vi "transfer char run_subvi_05_11a_JW.vi"(0 "VISA session":refnum<visa-resource-name>="GPIB0::17::INSTR", 5 "Var1 sweep settings":T4={"start"=40.0, "stop"=-40.0, "step (linear only)"=-1.0, "sweep spacing (linear: 0)"=0, "sweep mode"=FALSE, "compliance (V)"=100.0, "compliance (A)"=0.001} {"compliance (A)" format="%^.2e"; "compliance (V)" format="%.2f"; "sweep spacing (linear: 0)" items=["linear", "log 10", "log 25", "log 50"]; "step (linear only)" format="%.2f"; "stop" format="%.2f"; "start" format="%.2f"}, 7 "Var2 step settings":T3={"compliance (A)"=0.001, "compliance (V)"=100.0, "start"=-2.0, "total points"=2, "step"=-38.0} {"step" format="%.2f"; "start" format="%.2f"; "compliance (V)" format="%.2f"; "compliance (A)" format="%^.2e"}, 9 "integration time":u32(slide) scale=0.0..2.0, 11 "Input Path":path, 13 "Sample Properties:":T1 {"Date Created" format="%<%x>T"}) -> (1 "Trap Density-STS":dbl, 3 "Trap Density-VT":dbl, 4 "Mobility":dbl, 6 "graphic display":cluster{"trace":dbl[], "trace":dbl[]}(graph), 8 "On/Off Current":dbl, 10 "XY Graph":cluster{dbl[], "trace":dbl[]}[](graph), 12 "Vt":dbl, 14 "STS":dbl, 15 "error?":errorcluster)   [LabVIEW 2011]
uses:
  <vilib>/Utility/file.llb/Write To Spreadsheet File (DBL).vi
  <vilib>/Utility/file.llb/Read From Spreadsheet File (string).vi
  <vilib>/Utility/file.llb/Write To Spreadsheet File (string).vi
  <vilib>/Analysis/NI_AALPro.lvlib
panel:
  out "Array":string[][](array[string])
  in  "Output Path":path
  in  "Temp (K)":dbl=0.001 format="%^.2e"
  in  "NumPts":dbl=5.0
  out "Numeric":dbl
  out "Max R":i32[](listbox)
  out "min r":dbl
  out "max r":dbl
  out "error? 2":errorcluster
  in  "MAXIMUM":ext format="%.2e"
  in  "MINIMUM":ext=-1e-05 format="%_2e"
  out "graphic display 2":cluster{"trace":dbl[], "trace":dbl[]}(graph)
  in  "Y1 axis":string="Id"
  in  "Y2 axis settings":T2 {"MAXIMUM" format="%.9f"; "MINIMUM" format="%.9f"}
  in  "wait time parameter":dbl=1.0
  in  "Value (Either V or A) 4":dbl
  in  "Value (Either V or A) 3":dbl
  in  "Value (Either V or A) 2":dbl
  in  "Value (V or A)":dbl
  in  "compliance (A)":dbl=0.001 format="%^.2e"
  in  "compliance (V)":dbl=100.0 format="%^.2e"
  in  "Iname":string="Is"
  in  "Vname":string="Vs"
  in  "Function":u16(ring)=4 items=["disabled", "Var1", "Var2", "Var1'", "Constant"]
  in  "Mode":u16(ring)=4 items=["V", "I", "VPulse", "IPulse", "Common"]
  in  "Iname 4":string="I4"
  in  "Vname 4":string="V4"
  in  "Function 4":u16(ring)=4 items=["disabled", "Var1", "Var2", "Var1'", "Constant"]
  in  "Mode 4":u16(ring) items=["V", "I", "VPulse", "IPulse", "Common"]
  in  "Iname 3":string="Ig"
  in  "Vname 3":string="Vg"
  in  "Function 3":u16(ring)=1 items=["disabled", "Var1", "Var2", "Var1'", "Constant"]
  in  "Mode 3":u16(ring) items=["V", "I", "VPulse", "IPulse", "Common"]
  in  "Iname 2":string="Id"
  in  "Vname 2":string="Vd"
  in  "Function 2":u16(ring)=2 items=["disabled", "Var1", "Var2", "Var1'", "Constant"]
  in  "Mode 2":u16(ring) items=["V", "I", "VPulse", "IPulse", "Common"]
  in  "reset":bool=TRUE
  # "SMU1"
  # "SMU2"
  # "SMU3"
  # "SMU4"
  # "Sample Properties:"
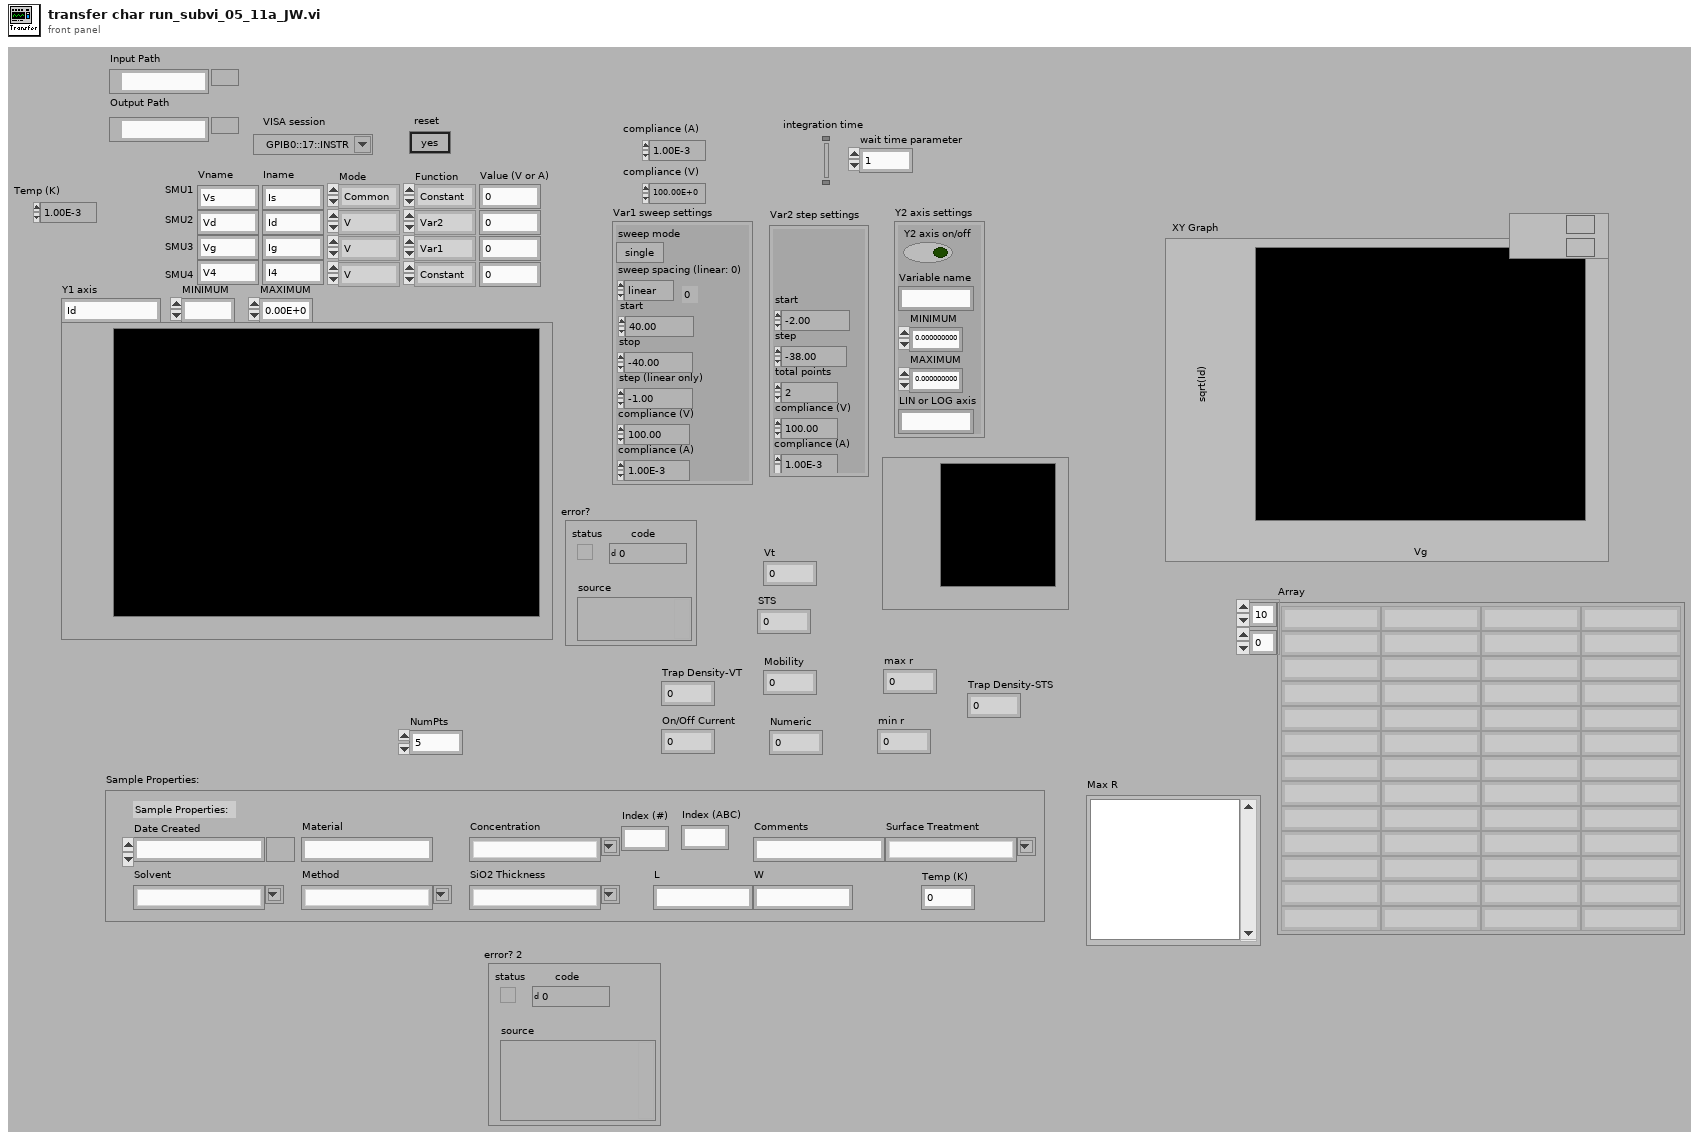
[diagram p1: front panel]
types:
  T1 = cluster{"Date Created":timestamp, "Material":string, "Solvent":string, "Concentration":string, "Method":string, "SiO2 Thickness":string, "Index (#)":string, "Index (ABC)":string, "L":string, "W":string, "Surface Treatment":string, "Comments":string, "Temp (K)":dbl}
  T2 = cluster{"Y2 axis on/off":bool, "MINIMUM":ext, "MAXIMUM":ext, "Variable name":string, "LIN or LOG axis":string}
  T3 = cluster{"compliance (A)":dbl, "compliance (V)":dbl, "start":dbl, "total points":u16, "step":dbl}
  T4 = cluster{"start":dbl, "stop":dbl, "step (linear only)":dbl, "sweep spacing (linear: 0)":u16, "sweep mode":bool, "compliance (V)":dbl, "compliance (A)":dbl}
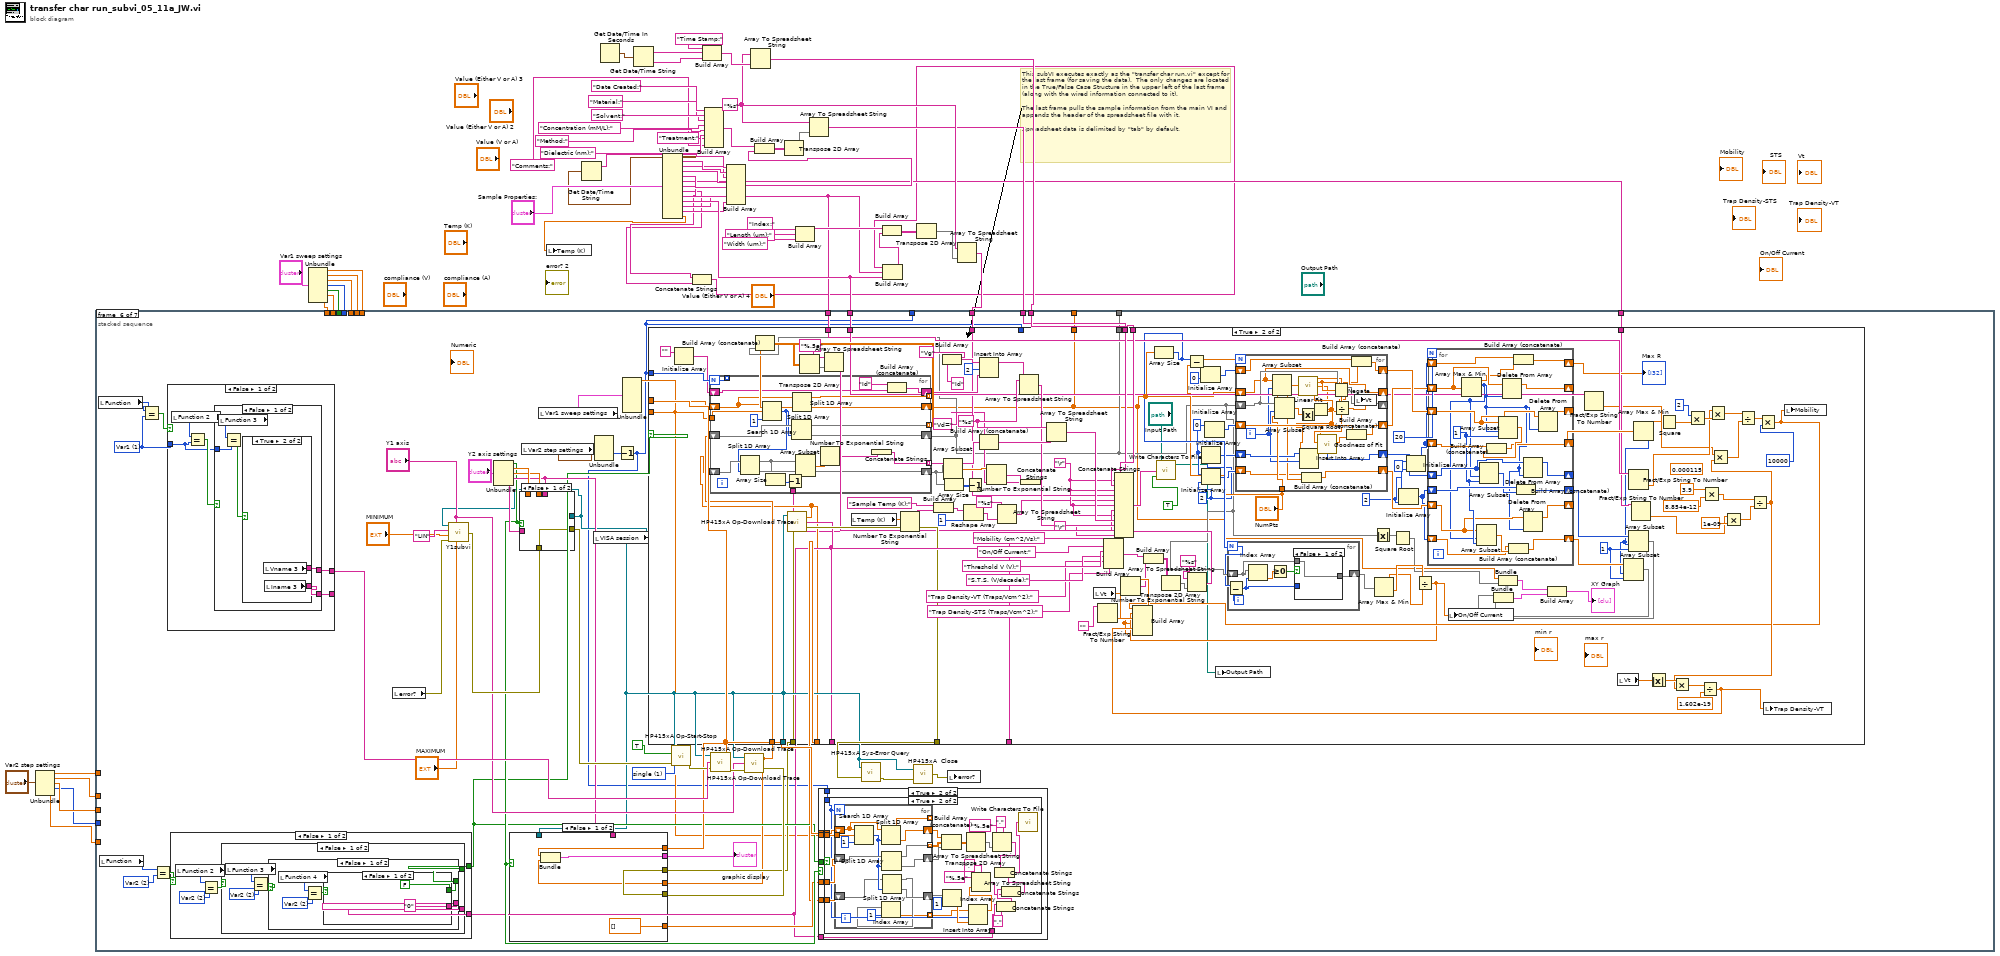
[diagram p0: block diagram]
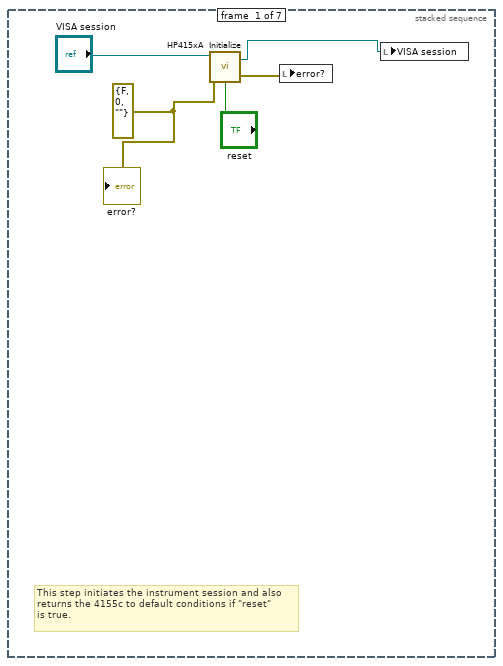
[diagram p2: hidden frame]
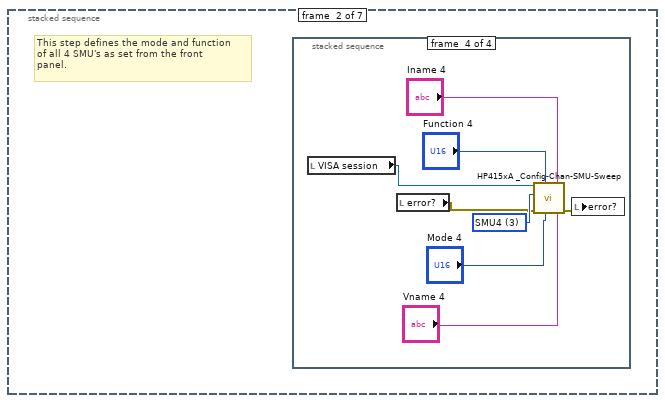
[diagram p3: hidden frame]
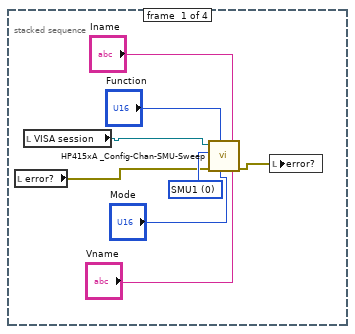
[diagram p4: hidden frame]
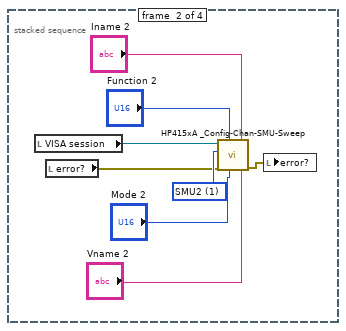
[diagram p5: hidden frame]
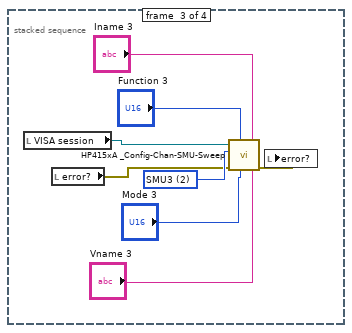
[diagram p6: hidden frame]
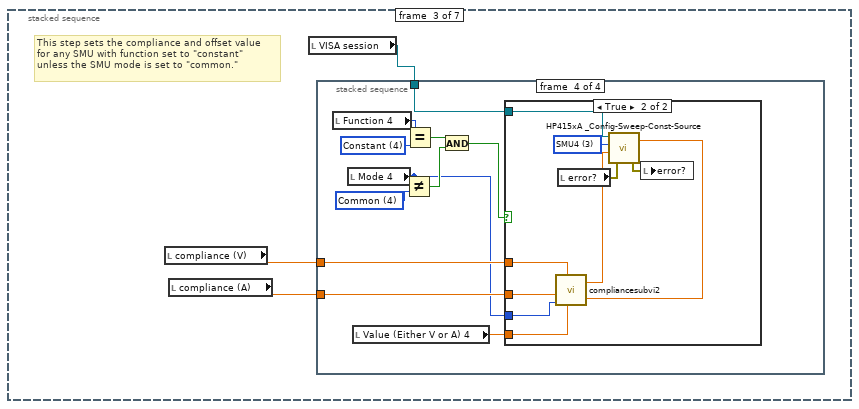
[diagram p7: hidden frame]
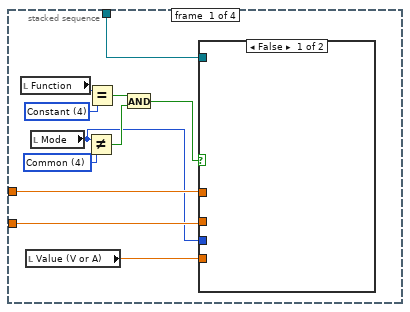
[diagram p8: hidden frame]
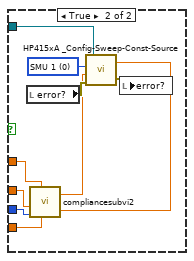
[diagram p9: hidden frame]
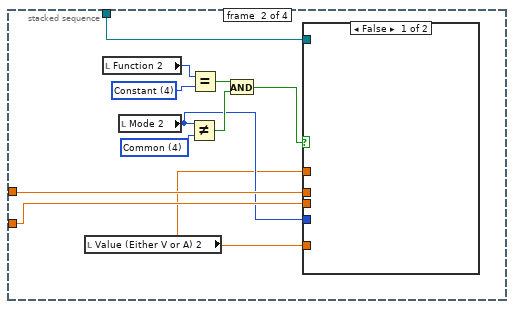
[diagram p10: hidden frame]
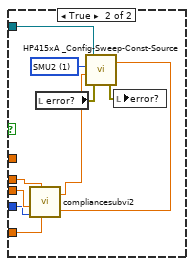
[diagram p11: hidden frame]
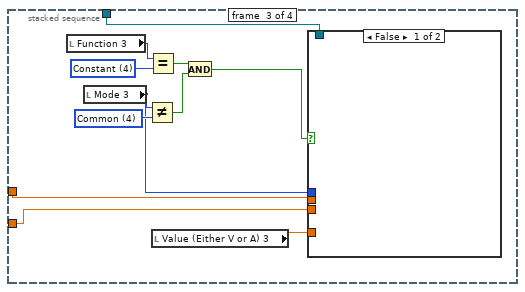
[diagram p12: hidden frame]
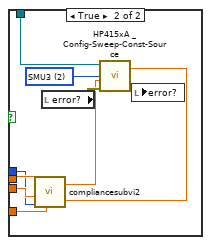
[diagram p13: hidden frame]
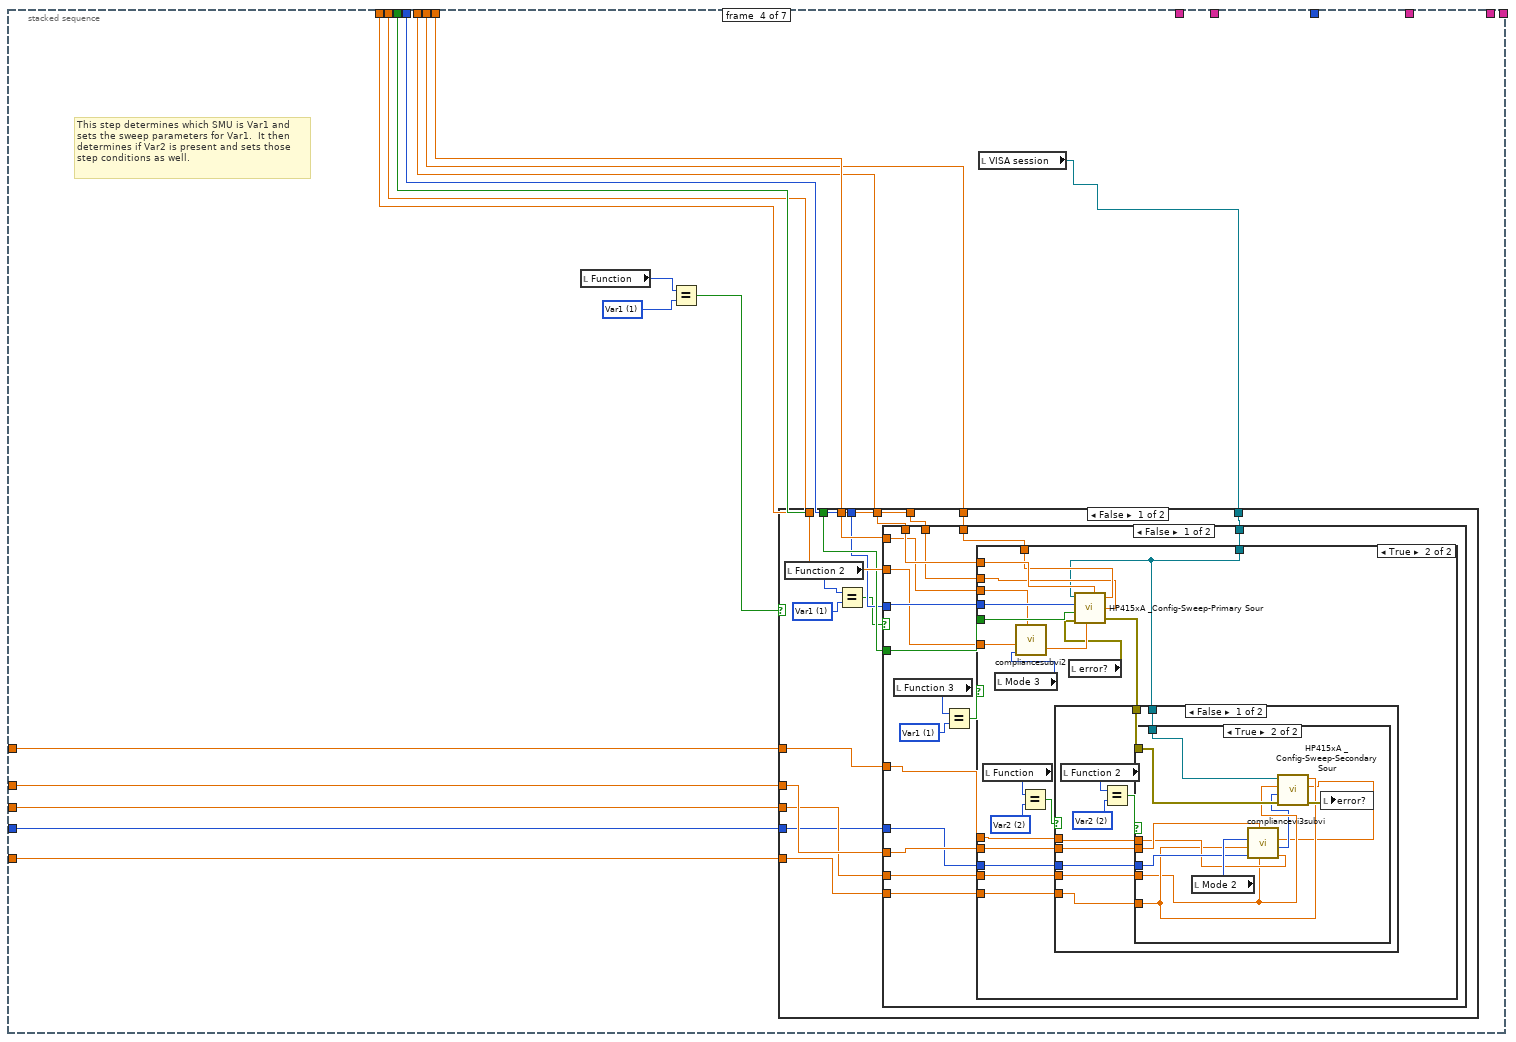
[diagram p15: hidden frame]
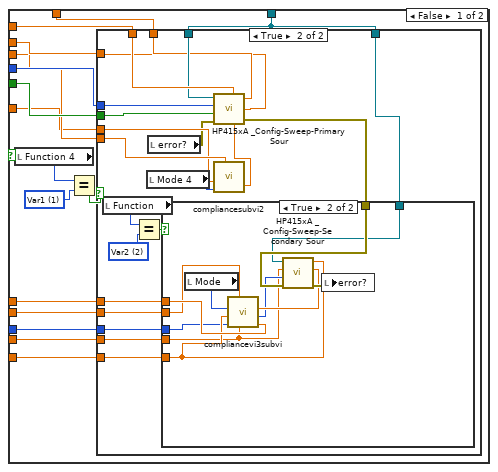
[diagram p16: hidden frame]
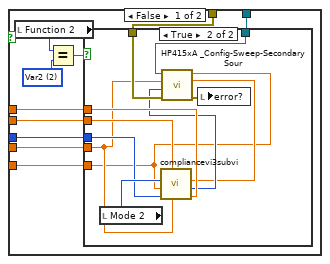
[diagram p18: hidden frame]
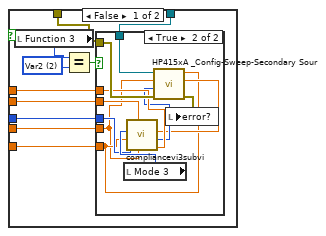
[diagram p19: hidden frame]
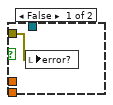
[diagram p20: hidden frame]
diagram:
  w31 = "%s"
  # "This subVI executes exactly as the \"transfer char run.vi\" except for the last frame (for saving the data).  The only changes are located in the True/False Case Structure in the upper left of the last frame (along with the wired information connected to it). \n\nThe last frame pulls the sample information from the main VI and appends the header of the spreadsheet file with it.\n\nSpreadsheet data is delimited by \"tab\" by default."
  n1 = Unbundle("Var2 step settings") -> ("compliance (A)"=w49:dbl, "compliance (V)"=w48:dbl, "start"=w47:dbl, "total points"=w46:u16, "step"=w45:dbl)
  n2 = Unbundle("Var1 sweep settings") -> ("start"=w57:dbl, "stop"=w56:dbl, "step (linear only)"=w55:dbl, "sweep spacing (linear: 0)"=w54:u16, "sweep mode"=w53:bool, "compliance (V)"=w52:dbl, "compliance (A)"=w51:dbl)
  n3 = Get Date/Time In Seconds() -> (seconds since 1Jan1904=w38:timestamp)
  n4 = Get Date/Time String(seconds (now)=w38) -> (date string=w37:string, time string=w36:string)  [unwired: 2 in]
  n5 = Unbundle("Sample Properties:") -> ("Date Created"=w16:timestamp, "Material"=w15:string, "Solvent"=w11:string, "Concentration"=w10:string, "Method"=w14:string, "SiO2 Thickness"=w9:string, "Index (#)"=w4:string, "Index (ABC)"=w3:string, "L"=w7:string, "W"=w8:string, "Surface Treatment"=w6:string, "Comments"=w5:string, "Temp (K)"=w1:dbl)
  n6 = local write "Temp (K)"(w1) -> ()
  n7 = Get Date/Time String(seconds (now)=w16) -> (date string=w43:string)  [unwired: 2 in, 1 out]
  n8 = Concatenate Strings(w4, w3) -> (w2:string)
  n9 = Build Array("Time Stamp:", w37, w36) -> (w35:string[])
  n10 = Build Array("Date Created:", "Material:", "Solvent:", "Concentration (mM/L):", "Method:", "Dielectric (nm):", "Treatment:", "Comments:") -> (w26:string[])
  n11 = Build Array(w43, w15, w11, w10, w14, w9, w6, w5) -> (w25:string[])
  n12 = Array To Spreadsheet String(array=w35, 3:w31) -> (spreadsheet string=w27:string)  [unwired: 1 in]
  n13 = Build Array(w26, w25) -> (w24:string[][])
  n14 = Transpose 2D Array(2D array=w24) -> (transposed array=w23:string[][])
  n15 = Build Array("Index:", "Length (um):", "Width (um):") -> (w22:string[])
  n16 = Array To Spreadsheet String(array=w23, 3:w31) -> (spreadsheet string=w30:string)  [unwired: 1 in]
  n17 = Build Array(w2, w7, w8) -> (w21:string[])
  n18 = Build Array(w22, w21) -> (w20:string[][])
  n19 = Transpose 2D Array(2D array=w20) -> (transposed array=w19:string[][])
  n20 = Array To Spreadsheet String(array=w19, 3:w31) -> (spreadsheet string=w18:string)  [unwired: 1 in]
  n21 = stacked-sequence {
    tunnel: w57 -> [_ _ _ w194 _ _ _]
    tunnel: w56 -> [_ _ _ w193 _ _ _]
    tunnel: w55 -> [_ _ _ w192 _ _ _]
    tunnel: w54 -> [_ _ _ w191 _ _ _]
    tunnel: w53 -> [_ _ _ w190 _ _ _]
    tunnel: w52 -> [_ _ _ w189 _ _ _]
    tunnel: w51 -> [_ _ _ w188 _ _ _]
    tunnel: w49 -> [_ _ _ w187 _ _ _]
    tunnel: w48 -> [_ _ _ w186 _ _ _]
    tunnel: w47 -> [_ _ _ w185 _ _ _]
    tunnel: w46 -> [_ _ _ w184 _ _ _]
    tunnel: w45 -> [_ _ _ w183 _ _ _]
    tunnel: w27 -> [_ _ _ _ _ w557 _]
    tunnel: w30 -> [_ _ _ _ _ w556 _]
    tunnel: w18 -> [_ _ _ _ _ w555 _]
    tunnel: [_ _ _ _ _ w554 _] -> _
    tunnel: [_ _ _ _ _ w553 _] -> _
    tunnel: [_ _ _ _ _ w550 _] -> _
    tunnel: w8 -> [_ _ _ _ _ w552 _]
    tunnel: w7 -> [_ _ _ _ _ w551 _]
    tunnel: w9 -> [_ _ _ _ _ w549 _]
    frame #0 {
      w62 = errorcluster {"status"=FALSE, "code"=0, "source"=""} ("error out")
      # "This step initiates the instrument session and also\nreturns the 4155c to default conditions if \"reset\"\nis true."
      n22 = call "HP415xA  Initialize.vi"("instrument descriptor"="VISA session", "reset"="reset", "error in (no error)"=w62) -> ("VISA session"=w59:refnum<visa-resource-name>, "error out"=w61:errorcluster)  [unwired: 2 in]
      n23 = local write "error?"(w61) -> ()
      n24 = local write "VISA session"(w59) -> ()
      "error?" <- w62
    }
    frame #1 {
      # "This step defines the mode and function\nof all 4 SMU's as set from the front\npanel."
      n25 = stacked-sequence {
        frame #0 {
          w71 = u32 0 items=["SMU1  ", "SMU2  ", "SMU3  ", "SMU4  ", "SMU5  ", "SMU6  "] ("unit to configure")
          n26 = local read "error?"() -> (w66:errorcluster)
          n27 = local read "VISA session"() -> (w64:refnum<visa-resource-name>)
          n28 = call "HP415xA _Config-Chan-SMU-Sweep.vi"("V name (max 6 chars)"="Vname", "I name (max 6 chars)"="Iname", "mode"="Mode", "function"="Function", "error in (no error)"=w66, "unit to configure"=w71, "VISA session"=w64) -> ("error out"=w65:errorcluster)  [unwired: 2 in]
          n29 = local write "error?"(w65) -> ()
        }
        frame #1 {
          w75 = u32 1 items=["SMU1  ", "SMU2  ", "SMU3  ", "SMU4  ", "SMU5  ", "SMU6  "] ("unit to configure")
          n30 = local read "VISA session"() -> (w72:refnum<visa-resource-name>)
          n31 = local read "error?"() -> (w73:errorcluster)
          n32 = call "HP415xA _Config-Chan-SMU-Sweep.vi"("V name (max 6 chars)"="Vname 2", "I name (max 6 chars)"="Iname 2", "mode"="Mode 2", "function"="Function 2", "error in (no error)"=w73, "unit to configure"=w75, "VISA session"=w72) -> ("error out"=w74:errorcluster)  [unwired: 2 in]
          n33 = local write "error?"(w74) -> ()
        }
        frame #2 {
          w83 = u32 2 items=["SMU1  ", "SMU2  ", "SMU3  ", "SMU4  ", "SMU5  ", "SMU6  "] ("unit to configure")
          n34 = local read "VISA session"() -> (w80:refnum<visa-resource-name>)
          n35 = local read "error?"() -> (w81:errorcluster)
          n36 = call "HP415xA _Config-Chan-SMU-Sweep.vi"("V name (max 6 chars)"="Vname 3", "I name (max 6 chars)"="Iname 3", "mode"="Mode 3", "function"="Function 3", "error in (no error)"=w81, "unit to configure"=w83, "VISA session"=w80) -> ("error out"=w82:errorcluster)  [unwired: 2 in]
          n37 = local write "error?"(w82) -> ()
        }
        frame #3 {
          w91 = u32 3 items=["SMU1  ", "SMU2  ", "SMU3  ", "SMU4  ", "SMU5  ", "SMU6  "] ("unit to configure")
          n38 = local read "VISA session"() -> (w88:refnum<visa-resource-name>)
          n39 = local read "error?"() -> (w90:errorcluster)
          n40 = call "HP415xA _Config-Chan-SMU-Sweep.vi"("V name (max 6 chars)"="Vname 4", "I name (max 6 chars)"="Iname 4", "mode"="Mode 4", "function"="Function 4", "error in (no error)"=w90, "unit to configure"=w91, "VISA session"=w88) -> ("error out"=w89:errorcluster)  [unwired: 2 in]
          n41 = local write "error?"(w89) -> ()
        }
      }
    }
    frame #2 {
      # "This step sets the compliance and offset value\nfor any SMU with function set to \"constant\"\nunless the SMU mode is set to \"common.\""
      n42 = local read "compliance (V)"() -> (w97:dbl)
      n43 = local read "compliance (A)"() -> (w98:dbl)
      n44 = local read "VISA session"() -> (w96:refnum<visa-resource-name>)
      n45 = stacked-sequence {
        tunnel: w96 -> [w107 w127 w146 w166]
        tunnel: w98 -> [w101 w123 w144 w164]
        tunnel: w97 -> [w100 w122 w143 w165]
        frame #0 {
          w105 = u16 4 items=["V", "I", "VPulse", "IPulse", "Common"] ("Mode")
          w109 = u16 4 items=["disabled", "Var1", "Var2", "Var1'", "Constant"] ("Function")
          n46 = local read "Function"() -> (w108:u16)
          n47 = local read "Value (V or A)"() -> (w102:dbl)
          n48 = local read "Mode"() -> (w99:u16)
          n49 = Not Equal?(x=w99, y=w105) -> (x != y?=w104:bool)
          n50 = Equal?(x=w108, y=w109) -> (x = y?=w106:bool)
          n51 = And(x=w106, y=w104) -> (x .and. y?=w103:bool)
          n52 = case shown="False" w103 {
            tunnel: w107 -> [_ w119]
            tunnel: w100 -> [_ w115]
            tunnel: w101 -> [_ w114]
            tunnel: w102 -> [_ w111]
            tunnel: w99 -> [_ w112]
            frame False {
            }
            frame True {
              w118 = u16 0 items=["SMU 1", "SMU2", "SMU3", "SMU4", "SMU5", "SMU6", "VSU1", "VSU2"] ("unit (SMU1:0)")
              n53 = local read "error?"() -> (w117:errorcluster)
              n54 = call "compliancesubvi2.vi"("Value1"=w111, "compliance (V)"=w115, "Mode"=w112, "compliance (A)"=w114) -> ("compliance"=w113:dbl, "constant"=w110:dbl)  [unwired: 2 in]
              n55 = call "HP415xA _Config-Sweep-Const-Source.vi"("compliance (SMUs only)"=w113, "error in (no error)"=w117, "source (V or A)"=w110, "unit (SMU1:0)"=w118, "VISA session"=w119) -> ("error out"=w116:errorcluster)
              n56 = local write "error?"(w116) -> ()
            }
          }
        }
        frame #1 {
          w124 = u16 4 items=["V", "I", "VPulse", "IPulse", "Common"] ("Mode 2")
          w125 = u16 4 items=["disabled", "Var1", "Var2", "Var1'", "Constant"] ("Function 2")
          n57 = local read "Value (Either V or A) 2"() -> (w120:dbl)
          n58 = local read "Function 2"() -> (w126:u16)
          n59 = local read "Mode 2"() -> (w121:u16)
          n60 = Not Equal?(x=w121, y=w124) -> (x != y?=w129:bool)
          n61 = Equal?(x=w126, y=w125) -> (x = y?=w130:bool)
          n62 = And(x=w130, y=w129) -> (x .and. y?=w128:bool)
          n63 = case shown="False" w128 {
            tunnel: w127 -> [_ w140]
            tunnel: w122 -> [_ w138]
            tunnel: w123 -> [_ w137]
            tunnel: w120 -> [_ _]
            tunnel: w121 -> [_ w133]
            tunnel: w120 -> [_ w132]
            frame False {
            }
            frame True {
              w139 = u16 1 items=["SMU 1", "SMU2", "SMU3", "SMU4", "SMU5", "SMU6", "VSU1", "VSU2"] ("unit (SMU1:0)")
              n64 = call "compliancesubvi2.vi"("Value1"=w132, "compliance (V)"=w138, "Mode"=w133, "compliance (A)"=w137) -> ("compliance"=w136:dbl, "constant"=w131:dbl)  [unwired: 2 in]
              n65 = local read "error?"() -> (w135:errorcluster)
              n66 = call "HP415xA _Config-Sweep-Const-Source.vi"("compliance (SMUs only)"=w136, "error in (no error)"=w135, "source (V or A)"=w131, "unit (SMU1:0)"=w139, "VISA session"=w140) -> ("error out"=w134:errorcluster)
              n67 = local write "error?"(w134) -> ()
            }
          }
        }
        frame #2 {
          w148 = u16 4 items=["V", "I", "VPulse", "IPulse", "Common"] ("Mode 2")
          w149 = u16 4 items=["disabled", "Var1", "Var2", "Var1'", "Constant"] ("Function 2")
          n68 = local read "Function 3"() -> (w147:u16)
          n69 = local read "Mode 3"() -> (w142:u16)
          n70 = Not Equal?(x=w142, y=w148) -> (x != y?=w150:bool)
          n71 = Equal?(x=w147, y=w149) -> (x = y?=w151:bool)
          n72 = local read "Value (Either V or A) 3"() -> (w145:dbl)
          n73 = And(x=w151, y=w150) -> (x .and. y?=w141:bool)
          n74 = case shown="False" w141 {
            tunnel: w146 -> [_ w159]
            tunnel: w145 -> [_ w153]
            tunnel: w144 -> [_ w156]
            tunnel: w143 -> [_ w155]
            tunnel: w142 -> [_ w154]
            frame False {
            }
            frame True {
              w158 = u16 2 items=["SMU 1", "SMU2", "SMU3", "SMU4", "SMU5", "SMU6", "VSU1", "VSU2"] ("unit (SMU1:0)")
              n75 = call "compliancesubvi2.vi"("Value1"=w153, "compliance (V)"=w155, "Mode"=w154, "compliance (A)"=w156) -> ("compliance"=w157:dbl, "constant"=w152:dbl)  [unwired: 2 in]
              n76 = local read "error?"() -> (w161:errorcluster)
              n77 = call "HP415xA _Config-Sweep-Const-Source.vi"("compliance (SMUs only)"=w157, "error in (no error)"=w161, "source (V or A)"=w152, "unit (SMU1:0)"=w158, "VISA session"=w159) -> ("error out"=w160:errorcluster)
              n78 = local write "error?"(w160) -> ()
            }
          }
        }
        frame #3 {
          w168 = u16 4 items=["V", "I", "VPulse", "IPulse", "Common"] ("Mode 4")
          w169 = u16 4 items=["disabled", "Var1", "Var2", "Var1'", "Constant"] ("Function 4")
          n79 = local read "Function 4"() -> (w170:u16)
          n80 = local read "Mode 4"() -> (w163:u16)
          n81 = local read "Value (Either V or A) 4"() -> (w162:dbl)
          n82 = Not Equal?(x=w163, y=w168) -> (x != y?=w171:bool)
          n83 = Equal?(x=w170, y=w169) -> (x = y?=w172:bool)
          n84 = And(x=w172, y=w171) -> (x .and. y?=w167:bool)
          n85 = case shown="True" w167 {
            tunnel: w166 -> [_ w181]
            tunnel: w165 -> [_ w177]
            tunnel: w164 -> [_ w178]
            tunnel: w163 -> [_ w176]
            tunnel: w162 -> [_ w175]
            frame False {
            }
            frame True {
              w182 = u16 3 items=["SMU 1", "SMU2", "SMU3", "SMU4", "SMU5", "SMU6", "VSU1", "VSU2"] ("unit (SMU1:0)")
              n86 = call "compliancesubvi2.vi"("Value1"=w175, "compliance (V)"=w177, "Mode"=w176, "compliance (A)"=w178) -> ("compliance"=w174:dbl, "constant"=w173:dbl)  [unwired: 2 in]
              n87 = local read "error?"() -> (w180:errorcluster)
              n88 = call "HP415xA _Config-Sweep-Const-Source.vi"("compliance (SMUs only)"=w174, "error in (no error)"=w180, "source (V or A)"=w173, "unit (SMU1:0)"=w182, "VISA session"=w181) -> ("error out"=w179:errorcluster)
              n89 = local write "error?"(w179) -> ()
            }
          }
        }
      }
    }
    frame #3 {
      w198 = u16 1 items=["disabled", "Var1", "Var2", "Var1'", "Constant"] ("Function")
      # "This step determines which SMU is Var1 and\nsets the sweep parameters for Var1.  It then\ndetermines if Var2 is present and sets those\nstep conditions as well."
      n90 = local read "Function"() -> (w197:u16)
      n91 = Equal?(x=w197, y=w198) -> (x = y?=w196:bool)
      n92 = local read "VISA session"() -> (w195:refnum<visa-resource-name>)
      n93 = case shown="False" w196 {
        tunnel: w189 -> [w211 w487]
        tunnel: w188 -> [w212 w486]
        tunnel: w191 -> [w209 w485]
        tunnel: w190 -> [w210 w484]
        tunnel: w192 -> [w206 w483]
        tunnel: w193 -> [w205 w482]
        tunnel: w194 -> [w207 w481]
        tunnel: w195 -> [w208 w470]
        tunnel: w187 -> [w203 w476]
        tunnel: w186 -> [w202 w475]
        tunnel: w185 -> [w201 w474]
        tunnel: w184 -> [w200 w473]
        tunnel: w183 -> [w199 w472]
        frame False {
          w214 = u16 1 items=["disabled", "Var1", "Var2", "Var1'", "Constant"] ("Function")
          n94 = local read "Function 2"() -> (w213:u16)
          n95 = Equal?(x=w213, y=w214) -> (x = y?=w204:bool)
          n96 = case shown="False" w204 {
            tunnel: w212 -> [w220 w413]
            tunnel: w211 -> [w221 w412]
            tunnel: w210 -> [w222 w411]
            tunnel: w209 -> [w223 w410]
            tunnel: w208 -> [w227 w399]
            tunnel: w207 -> [w226 w409]
            tunnel: w206 -> [w224 w408]
            tunnel: w205 -> [w225 w407]
            tunnel: w203 -> [w219 w402]
            tunnel: w202 -> [w218 w401]
            tunnel: w201 -> [w216 w400]
            tunnel: w200 -> [w217 w397]
            tunnel: w199 -> [w215 w396]
            frame False {
              w230 = u16 1 items=["disabled", "Var1", "Var2", "Var1'", "Constant"] ("Function")
              n97 = local read "Function 3"() -> (w229:u16)
              n98 = Equal?(x=w229, y=w230) -> (x = y?=w228:bool)
              n99 = case shown="True" w228 {
                tunnel: w227 -> [w231 w324]
                tunnel: w226 -> [w243 w341]
                tunnel: w225 -> [w240 w340]
                tunnel: w224 -> [w239 w339]
                tunnel: w223 -> [w242 w338]
                tunnel: w222 -> [w241 w337]
                tunnel: w221 -> [w238 w336]
                tunnel: w220 -> [w237 w335]
                tunnel: w219 -> [w236 w328]
                tunnel: w218 -> [w235 w327]
                tunnel: w217 -> [w234 w326]
                tunnel: w216 -> [w233 w323]
                tunnel: w215 -> [w232 w322]
                frame False {
                  w246 = u16 1 items=["disabled", "Var1", "Var2", "Var1'", "Constant"] ("Function")
                  n100 = local read "Function 4"() -> (w245:u16)
                  n101 = Equal?(x=w245, y=w246) -> (x = y?=w244:bool)
                  n102 = case shown="True" w244 {
                    tunnel: w243 -> [_ w265]
                    tunnel: w231 -> [_ w264]
                    tunnel: w242 -> [_ w263]
                    tunnel: w241 -> [_ w262]
                    tunnel: w240 -> [_ w261]
                    tunnel: w239 -> [_ w260]
                    tunnel: w238 -> [_ w259]
                    tunnel: w237 -> [_ w258]
                    tunnel: w236 -> [_ w253]
                    tunnel: w235 -> [_ w252]
                    tunnel: w234 -> [_ w251]
                    tunnel: w233 -> [_ w250]
                    tunnel: w232 -> [_ w249]
                    tunnel: w231 -> [_ w247]
                    frame False {
                    }
                    frame True {
                      w256 = u16 2 items=["disabled", "Var1", "Var2", "Var1'", "Constant"] ("Function")
                      n103 = local read "Function"() -> (w255:u16)
                      n104 = Equal?(x=w255, y=w256) -> (x = y?=w254:bool)
                      n105 = local read "Mode 4"() -> (w267:u16)
                      n106 = local read "error?"() -> (w257:errorcluster)
                      n107 = call "compliancesubvi2.vi"("compliance (V)"=w259, "Mode"=w267, "compliance (A)"=w258) -> ("compliance"=w266:dbl)  [unwired: 3 in, 1 out]
                      n108 = call "HP415xA _Config-Sweep-Primary Sour.vi"("step (linear only)"=w260, "stop"=w261, "start"=w265, "compliance"=w266, "error in (no error)"=w257, "sweep mode"=w262, "sweep spacing (linear: 0)"=w263, "VISA session"=w264) -> ("error out"=w248:errorcluster)  [unwired: 2 in]
                      n109 = case shown="True" w254 {
                        tunnel: w253 -> [w274 w317]
                        tunnel: w252 -> [w273 w312]
                        tunnel: w251 -> [w272 w311]
                        tunnel: w250 -> [w271 w313]
                        tunnel: w249 -> [w270 w316]
                        tunnel: w248 -> [w269 w319]
                        tunnel: w247 -> [w268 w318]
                        frame False {
                          w277 = u16 2 items=["disabled", "Var1", "Var2", "Var1'", "Constant"] ("Function")
                          n110 = local read "Function 2"() -> (w276:u16)
                          n111 = Equal?(x=w276, y=w277) -> (x = y?=w275:bool)
                          n112 = case shown="True" w275 {
                            tunnel: w274 -> [w285 w305]
                            tunnel: w273 -> [w284 w306]
                            tunnel: w272 -> [w283 w304]
                            tunnel: w271 -> [w282 w302]
                            tunnel: w270 -> [w281 w300]
                            tunnel: w269 -> [w280 w310]
                            tunnel: w268 -> [w278 w309]
                            frame False {
                              w287 = u16 2 items=["disabled", "Var1", "Var2", "Var1'", "Constant"] ("Function")
                              n113 = local read "Function 3"() -> (w279:u16)
                              n114 = Equal?(x=w279, y=w287) -> (x = y?=w286:bool)
                              n115 = case shown="True" w286 {
                                tunnel: w285 -> [_ w293]
                                tunnel: w284 -> [_ w294]
                                tunnel: w283 -> [_ w295]
                                tunnel: w282 -> [_ w289]
                                tunnel: w281 -> [_ w290]
                                tunnel: w280 -> [w288 w299]
                                tunnel: w278 -> [_ w298]
                                frame False {
                                n116 = local write "error?"(w288) -> ()
                                }
                                frame True {
                                n117 = local read "Mode 3"() -> (w297:u16)
                                n118 = call "compliancevi3subvi.vi"("compliance (A)"=w293, "start"=w289, "compliance (V)"=w294, "total points"=w295, "step"=w290, "Mode"=w297) -> ("total points 2"=w292:u16, "compliance"=w291:dbl)  [unwired: 1 in, 1 out]
                                n119 = call "HP415xA _Config-Sweep-Secondary Sour.vi"("compliance"=w291, "step"=w290, "error in (no error)"=w299, "total points"=w292, "start"=w289, "VISA session"=w298) -> ("error out"=w296:errorcluster)  [unwired: 1 in]
                                n120 = local write "error?"(w296) -> ()
                                }
                              }
                            }
                            frame True {
                              n121 = local read "Mode 2"() -> (w308:u16)
                              n122 = call "compliancevi3subvi.vi"("compliance (A)"=w305, "start"=w302, "compliance (V)"=w306, "total points"=w304, "step"=w300, "Mode"=w308) -> ("total points 2"=w303:u16, "compliance"=w301:dbl)  [unwired: 1 in, 1 out]
                              n123 = call "HP415xA _Config-Sweep-Secondary Sour.vi"("compliance"=w301, "step"=w300, "error in (no error)"=w310, "total points"=w303, "start"=w302, "VISA session"=w309) -> ("error out"=w307:errorcluster)  [unwired: 1 in]
                              n124 = local write "error?"(w307) -> ()
                            }
                          }
                        }
                        frame True {
                          n125 = local read "Mode"() -> (w321:u16)
                          n126 = call "compliancevi3subvi.vi"("compliance (A)"=w317, "start"=w313, "compliance (V)"=w312, "total points"=w311, "step"=w316, "Mode"=w321) -> ("total points 2"=w314:u16, "compliance"=w315:dbl)  [unwired: 1 in, 1 out]
                          n127 = call "HP415xA _Config-Sweep-Secondary Sour.vi"("compliance"=w315, "step"=w316, "error in (no error)"=w319, "total points"=w314, "start"=w313, "VISA session"=w318) -> ("error out"=w320:errorcluster)  [unwired: 1 in]
                          n128 = local write "error?"(w320) -> ()
                        }
                      }
                    }
                  }
                }
                frame True {
                  w331 = u16 2 items=["disabled", "Var1", "Var2", "Var1'", "Constant"] ("Function")
                  n129 = local read "Function"() -> (w330:u16)
                  n130 = local read "Mode 3"() -> (w333:u16)
                  n131 = call "compliancesubvi2.vi"("compliance (V)"=w336, "Mode"=w333, "compliance (A)"=w335) -> ("compliance"=w334:dbl)  [unwired: 3 in, 1 out]
                  n132 = Equal?(x=w330, y=w331) -> (x = y?=w329:bool)
                  n133 = local read "error?"() -> (w332:errorcluster)
                  n134 = call "HP415xA _Config-Sweep-Primary Sour.vi"("step (linear only)"=w339, "stop"=w340, "start"=w341, "compliance"=w334, "error in (no error)"=w332, "sweep mode"=w337, "sweep spacing (linear: 0)"=w338, "VISA session"=w324) -> ("error out"=w325:errorcluster)  [unwired: 2 in]
                  n135 = case shown="False" w329 {
                    tunnel: w328 -> [w346 w391]
                    tunnel: w327 -> [w345 w390]
                    tunnel: w326 -> [w343 w389]
                    tunnel: w325 -> [w348 w394]
                    tunnel: w324 -> [w347 w393]
                    tunnel: w323 -> [w342 w386]
                    tunnel: w322 -> [w344 w385]
                    frame False {
                      w351 = u16 2 items=["disabled", "Var1", "Var2", "Var1'", "Constant"] ("Function")
                      n136 = local read "Function 2"() -> (w350:u16)
                      n137 = Equal?(x=w350, y=w351) -> (x = y?=w349:bool)
                      n138 = case shown="True" w349 {
                        tunnel: w348 -> [w358 w383]
                        tunnel: w347 -> [w357 w382]
                        tunnel: w346 -> [w356 w378]
                        tunnel: w345 -> [w355 w379]
                        tunnel: w344 -> [w352 w377]
                        tunnel: w343 -> [w354 w380]
                        tunnel: w342 -> [w353 w376]
                        frame False {
                          w361 = u16 2 items=["disabled", "Var1", "Var2", "Var1'", "Constant"] ("Function")
                          n139 = local read "Function 4"() -> (w360:u16)
                          n140 = Equal?(x=w360, y=w361) -> (x = y?=w359:bool)
                          n141 = case shown="True" w359 {
                            tunnel: w358 -> [w362 w371]
                            tunnel: w357 -> [_ w372]
                            tunnel: w356 -> [_ w368]
                            tunnel: w355 -> [_ w369]
                            tunnel: w354 -> [_ w367]
                            tunnel: w353 -> [_ w364]
                            tunnel: w352 -> [_ w363]
                            frame False {
                              n142 = local write "error?"(w362) -> ()
                            }
                            frame True {
                              n143 = local read "Mode 4"() -> (w373:u16)
                              n144 = call "compliancevi3subvi.vi"("compliance (A)"=w368, "start"=w364, "compliance (V)"=w369, "total points"=w367, "step"=w363, "Mode"=w373) -> ("total points 2"=w366:u16, "compliance"=w365:dbl)  [unwired: 1 in, 1 out]
                              n145 = call "HP415xA _Config-Sweep-Secondary Sour.vi"("compliance"=w365, "step"=w363, "error in (no error)"=w371, "total points"=w366, "start"=w364, "VISA session"=w372) -> ("error out"=w370:errorcluster)  [unwired: 1 in]
                              n146 = local write "error?"(w370) -> ()
                            }
                          }
                        }
                        frame True {
                          n147 = local read "Mode 2"() -> (w384:u16)
                          n148 = call "compliancevi3subvi.vi"("compliance (A)"=w378, "start"=w376, "compliance (V)"=w379, "total points"=w380, "step"=w377, "Mode"=w384) -> ("total points 2"=w375:u16, "compliance"=w374:dbl)  [unwired: 1 in, 1 out]
                          n149 = call "HP415xA _Config-Sweep-Secondary Sour.vi"("compliance"=w374, "step"=w377, "error in (no error)"=w383, "total points"=w375, "start"=w376, "VISA session"=w382) -> ("error out"=w381:errorcluster)  [unwired: 1 in]
                          n150 = local write "error?"(w381) -> ()
                        }
                      }
                    }
                    frame True {
                      n151 = local read "Mode"() -> (w395:u16)
                      n152 = call "compliancevi3subvi.vi"("compliance (A)"=w391, "start"=w386, "compliance (V)"=w390, "total points"=w389, "step"=w385, "Mode"=w395) -> ("total points 2"=w388:u16, "compliance"=w387:dbl)  [unwired: 1 in, 1 out]
                      n153 = call "HP415xA _Config-Sweep-Secondary Sour.vi"("compliance"=w387, "step"=w385, "error in (no error)"=w394, "total points"=w388, "start"=w386, "VISA session"=w393) -> ("error out"=w392:errorcluster)  [unwired: 1 in]
                      n154 = local write "error?"(w392) -> ()
                    }
                  }
                }
              }
            }
            frame True {
              w405 = u16 2 items=["disabled", "Var1", "Var2", "Var1'", "Constant"] ("Function")
              n155 = local read "Mode 2"() -> (w414:u16)
              n156 = local read "Function"() -> (w404:u16)
              n157 = Equal?(x=w404, y=w405) -> (x = y?=w403:bool)
              n158 = local read "error?"() -> (w406:errorcluster)
              n159 = call "compliancesubvi2.vi"("compliance (V)"=w412, "Mode"=w414, "compliance (A)"=w413) -> ("compliance"=w415:dbl)  [unwired: 3 in, 1 out]
              n160 = call "HP415xA _Config-Sweep-Primary Sour.vi"("step (linear only)"=w408, "stop"=w407, "start"=w409, "compliance"=w415, "error in (no error)"=w406, "sweep mode"=w411, "sweep spacing (linear: 0)"=w410, "VISA session"=w399) -> ("error out"=w398:errorcluster)  [unwired: 2 in]
              n161 = case shown="True" w403 {
                tunnel: w402 -> [w421 w464]
                tunnel: w401 -> [w420 w463]
                tunnel: w400 -> [w418 w459]
                tunnel: w399 -> [w423 w469]
                tunnel: w398 -> [w417 w468]
                tunnel: w397 -> [w419 w465]
                tunnel: w396 -> [w416 w461]
                frame False {
                  w425 = u16 2 items=["disabled", "Var1", "Var2", "Var1'", "Constant"] ("Function")
                  n162 = local read "Function 3"() -> (w424:u16)
                  n163 = Equal?(x=w424, y=w425) -> (x = y?=w422:bool)
                  n164 = case shown="True" w422 {
                    tunnel: w423 -> [w431 w457]
                    tunnel: w421 -> [w430 w454]
                    tunnel: w420 -> [w428 w452]
                    tunnel: w419 -> [w429 w453]
                    tunnel: w418 -> [w426 w450]
                    tunnel: w417 -> [w432 w456]
                    tunnel: w416 -> [w427 w448]
                    frame False {
                      w435 = u16 2 items=["disabled", "Var1", "Var2", "Var1'", "Constant"] ("Function")
                      n165 = local read "Function 4"() -> (w434:u16)
                      n166 = Equal?(x=w434, y=w435) -> (x = y?=w433:bool)
                      n167 = case shown="True" w433 {
                        tunnel: w432 -> [w436 w447]
                        tunnel: w431 -> [_ w446]
                        tunnel: w430 -> [_ w443]
                        tunnel: w429 -> [_ w444]
                        tunnel: w428 -> [_ w442]
                        tunnel: w427 -> [_ w438]
                        tunnel: w426 -> [_ w439]
                        frame False {
                          n168 = local write "error?"(w436) -> ()
                        }
                        frame True {
                          n169 = local read "Mode 4"() -> (w441:u16)
                          n170 = call "compliancevi3subvi.vi"("compliance (A)"=w443, "start"=w439, "compliance (V)"=w442, "total points"=w444, "step"=w438, "Mode"=w441) -> ("total points 2"=w440:u16, "compliance"=w437:dbl)  [unwired: 1 in, 1 out]
                          n171 = call "HP415xA _Config-Sweep-Secondary Sour.vi"("compliance"=w437, "step"=w438, "error in (no error)"=w447, "total points"=w440, "start"=w439, "VISA session"=w446) -> ("error out"=w445:errorcluster)  [unwired: 1 in]
                          n172 = local write "error?"(w445) -> ()
                        }
                      }
                    }
                    frame True {
                      n173 = local read "Mode 3"() -> (w458:u16)
                      n174 = call "compliancevi3subvi.vi"("compliance (A)"=w454, "start"=w450, "compliance (V)"=w452, "total points"=w453, "step"=w448, "Mode"=w458) -> ("total points 2"=w451:u16, "compliance"=w449:dbl)  [unwired: 1 in, 1 out]
                      n175 = call "HP415xA _Config-Sweep-Secondary Sour.vi"("compliance"=w449, "step"=w448, "error in (no error)"=w456, "total points"=w451, "start"=w450, "VISA session"=w457) -> ("error out"=w455:errorcluster)  [unwired: 1 in]
                      n176 = local write "error?"(w455) -> ()
                    }
                  }
                }
                frame True {
                  n177 = local read "Mode"() -> (w466:u16)
                  n178 = call "compliancevi3subvi.vi"("compliance (A)"=w464, "start"=w459, "compliance (V)"=w463, "total points"=w465, "step"=w461, "Mode"=w466) -> ("total points 2"=w460:u16, "compliance"=w462:dbl)  [unwired: 1 in, 1 out]
                  n179 = call "HP415xA _Config-Sweep-Secondary Sour.vi"("compliance"=w462, "step"=w461, "error in (no error)"=w468, "total points"=w460, "start"=w459, "VISA session"=w469) -> ("error out"=w467:errorcluster)  [unwired: 1 in]
                  n180 = local write "error?"(w467) -> ()
                }
              }
            }
          }
        }
        frame True {
          w478 = u16 2 items=["disabled", "Var1", "Var2", "Var1'", "Constant"] ("Function 2")
          n181 = local read "error?"() -> (w480:errorcluster)
          n182 = local read "Mode"() -> (w488:u16)
          n183 = local read "Function 2"() -> (w479:u16)
          n184 = call "compliancesubvi2.vi"("compliance (V)"=w487, "Mode"=w488, "compliance (A)"=w486) -> ("compliance"=w489:dbl)  [unwired: 3 in, 1 out]
          n185 = call "HP415xA _Config-Sweep-Primary Sour.vi"("step (linear only)"=w483, "stop"=w482, "start"=w481, "compliance"=w489, "error in (no error)"=w480, "sweep mode"=w484, "sweep spacing (linear: 0)"=w485, "VISA session"=w470) -> ("error out"=w471:errorcluster)  [unwired: 2 in]
          n186 = Equal?(x=w479, y=w478) -> (x = y?=w477:bool)
          n187 = case shown="True" w477 {
            tunnel: w476 -> [w495 w539]
            tunnel: w475 -> [w496 w538]
            tunnel: w474 -> [w493 w535]
            tunnel: w473 -> [w494 w537]
            tunnel: w472 -> [w492 w533]
            tunnel: w471 -> [w491 w542]
            tunnel: w470 -> [w490 w540]
            frame False {
              w499 = u16 2 items=["disabled", "Var1", "Var2", "Var1'", "Constant"] ("Function 2")
              n188 = local read "Function 3"() -> (w498:u16)
              n189 = Equal?(x=w498, y=w499) -> (x = y?=w497:bool)
              n190 = case shown="True" w497 {
                tunnel: w496 -> [w504 w522]
                tunnel: w495 -> [w505 w523]
                tunnel: w494 -> [w502 w528]
                tunnel: w493 -> [w503 w525]
                tunnel: w492 -> [w501 w524]
                tunnel: w491 -> [w506 w531]
                tunnel: w490 -> [w500 w529]
                frame False {
                  w509 = u16 2 items=["disabled", "Var1", "Var2", "Var1'", "Constant"] ("Function 2")
                  n191 = local read "Function 4"() -> (w508:u16)
                  n192 = Equal?(x=w508, y=w509) -> (x = y?=w507:bool)
                  n193 = case shown="True" w507 {
                    tunnel: w506 -> [w510 w521]
                    tunnel: w505 -> [_ w511]
                    tunnel: w504 -> [_ w512]
                    tunnel: w503 -> [_ w513]
                    tunnel: w502 -> [_ w518]
                    tunnel: w501 -> [_ w515]
                    tunnel: w500 -> [_ w519]
                    frame False {
                      n194 = local write "error?"(w510) -> ()
                    }
                    frame True {
                      n195 = local read "Mode 4"() -> (w517:u16)
                      n196 = call "compliancevi3subvi.vi"("compliance (A)"=w511, "start"=w513, "compliance (V)"=w512, "total points"=w518, "step"=w515, "Mode"=w517) -> ("total points 2"=w514:u16, "compliance"=w516:dbl)  [unwired: 1 in, 1 out]
                      n197 = call "HP415xA _Config-Sweep-Secondary Sour.vi"("compliance"=w516, "step"=w515, "error in (no error)"=w521, "total points"=w514, "start"=w513, "VISA session"=w519) -> ("error out"=w520:errorcluster)  [unwired: 1 in]
                      n198 = local write "error?"(w520) -> ()
                    }
                  }
                }
                frame True {
                  n199 = local read "Mode 3"() -> (w532:u16)
                  n200 = call "compliancevi3subvi.vi"("compliance (A)"=w523, "start"=w525, "compliance (V)"=w522, "total points"=w528, "step"=w524, "Mode"=w532) -> ("total points 2"=w527:u16, "compliance"=w526:dbl)  [unwired: 1 in, 1 out]
                  n201 = call "HP415xA _Config-Sweep-Secondary Sour.vi"("compliance"=w526, "step"=w524, "error in (no error)"=w531, "total points"=w527, "start"=w525, "VISA session"=w529) -> ("error out"=w530:errorcluster)  [unwired: 1 in]
                  n202 = local write "error?"(w530) -> ()
                }
              }
            }
            frame True {
              n203 = local read "Mode 2"() -> (w543:u16)
              n204 = call "compliancevi3subvi.vi"("compliance (A)"=w539, "start"=w535, "compliance (V)"=w538, "total points"=w537, "step"=w533, "Mode"=w543) -> ("total points 2"=w536:u16, "compliance"=w534:dbl)  [unwired: 1 in, 1 out]
              n205 = call "HP415xA _Config-Sweep-Secondary Sour.vi"("compliance"=w534, "step"=w533, "error in (no error)"=w542, "total points"=w536, "start"=w535, "VISA session"=w540) -> ("error out"=w541:errorcluster)  [unwired: 1 in]
              n206 = local write "error?"(w541) -> ()
            }
          }
        }
      }
    }
    frame #4 {
      # "This step sets the integration time."
      n207 = local read "VISA session"() -> (w544:refnum<visa-resource-name>)
      n208 = local read "error?"() -> (w548:errorcluster)
      n209 = call "HP415xA _Config-Meas-Timing.vi"("error in (no error)"=w548, "wait time parameter"="wait time parameter", "integration time"="integration time", "VISA session"=w544) -> ("error out"=w547:errorcluster)  [unwired: 2 in]
      n210 = local write "error?"(w547) -> ()
    }
    frame #5 {
      w584 = u32 1 items=["stop  ", "single  ", "single-append  ", "stress start  ", "continuous  ", "standby on  ", "standby off  ", "zero  "] ("function (stop:0)")
      w588 = u16 2 items=["disabled", "Var1", "Var2", "Var1'", "Constant"] ("Function")
      w593 = u16 1 items=["disabled", "Var1", "Var2", "Var1'", "Constant"] ("Function")
      n211 = local read "Function"() -> (w595:u16)
      n212 = local read "Function"() -> (w587:u16)
      n213 = Equal?(x=w595, y=w593) -> (x = y?=w594:bool)
      n214 = Equal?(x=w587, y=w588) -> (x = y?=w586:bool)
      n215 = case shown="False" w594 {
        tunnel: [w952 w967] -> w589
        tunnel: [w953 w966] -> _
        tunnel: w593 -> [w950 _]
        frame False {
          n216 = local read "Function 2"() -> (w954:u16)
          n217 = Equal?(x=w954, y=w950) -> (x = y?=w951:bool)
          n218 = case shown="False" w951 {
            tunnel: [w955 w965] -> w953
            tunnel: [w956 w964] -> w952
            tunnel: w950 -> [w959 _]
            frame False {
              n219 = local read "Function 3"() -> (w958:u16)
              n220 = Equal?(x=w958, y=w959) -> (x = y?=w957:bool)
              n221 = case shown="True" w957 {
                tunnel: [w961 w963] -> w956
                tunnel: [w960 w962] -> w955
                frame False {
                  n222 = local read "Vname 4"() -> (w961:string)
                  n223 = local read "Iname 4"() -> (w960:string)
                }
                frame True {
                  n224 = local read "Vname 3"() -> (w963:string)
                  n225 = local read "Iname 3"() -> (w962:string)
                }
              }
            }
            frame True {
              n226 = local read "Vname 2"() -> (w964:string)
              n227 = local read "Iname 2"() -> (w965:string)
            }
          }
        }
        frame True {
          n228 = local read "Vname"() -> (w967:string)
          n229 = local read "Iname"() -> (w966:string)
        }
      }
      n230 = case shown="False" w586 {
        tunnel: [w894 w947] -> w559
        tunnel: [w893 TRUE ("x = y?")] -> w565
        frame False {
          w897 = u16 2 items=["disabled", "Var1", "Var2", "Var1'", "Constant"] ("Function")
          n231 = local read "Function 2"() -> (w896:u16)
          n232 = Equal?(x=w896, y=w897) -> (x = y?=w895:bool)
          n233 = case shown="False" w895 {
            tunnel: [w899 w937] -> w894
            tunnel: [w898 TRUE ("x = y?")] -> w893
            frame False {
              w902 = u16 2 items=["disabled", "Var1", "Var2", "Var1'", "Constant"] ("Function")
              n234 = local read "Function 3"() -> (w901:u16)
              n235 = Equal?(x=w901, y=w902) -> (x = y?=w900:bool)
              n236 = case shown="False" w900 {
                tunnel: [w907 w927] -> w899
                tunnel: [w903 TRUE ("x = y?")] -> w898
                frame False {
                  w906 = u16 2 items=["disabled", "Var1", "Var2", "Var1'", "Constant"] ("Function")
                  n237 = local read "Function 4"() -> (w905:u16)
                  n238 = Equal?(x=w905, y=w906) -> (x = y?=w904:bool)
                  n239 = case shown="False" w904 {
                    tunnel: ["0" ("Vname 4") w917] -> w907
                    tunnel: [FALSE ("x = y?") TRUE ("x = y?")] -> w903
                    frame False {
                    }
                    frame True {
                      w911 = u16 2 items=["V", "I", "VPulse", "IPulse", "Common"] ("Mode 2")
                      w914 = u16 0 items=["V", "I", "VPulse", "IPulse", "Common"] ("Mode 2")
                      n240 = local read "Mode 4"() -> (w913:u16)
                      n241 = Equal?(x=w914, y=w913) -> (x = y?=w915:bool)
                      n242 = Equal?(x=w913, y=w911) -> (x = y?=w912:bool)
                      n243 = Or(x=w915, y=w912) -> (x .or. y?=w910:bool)
                      n244 = case shown="False" w910 {
                        tunnel: [w918 w919] -> w917
                        frame False {
                          n245 = local read "Iname 4"() -> (w918:string)
                        }
                        frame True {
                          n246 = local read "Vname 4"() -> (w919:string)
                        }
                      }
                    }
                  }
                }
                frame True {
                  w923 = u16 2 items=["V", "I", "VPulse", "IPulse", "Common"] ("Mode 2")
                  w922 = u16 0 items=["V", "I", "VPulse", "IPulse", "Common"] ("Mode 2")
                  n247 = local read "Mode 3"() -> (w921:u16)
                  n248 = Equal?(x=w922, y=w921) -> (x = y?=w925:bool)
                  n249 = Equal?(x=w921, y=w923) -> (x = y?=w924:bool)
                  n250 = Or(x=w925, y=w924) -> (x .or. y?=w920:bool)
                  n251 = case shown="False" w920 {
                    tunnel: [w928 w929] -> w927
                    frame False {
                      n252 = local read "Iname 3"() -> (w928:string)
                    }
                    frame True {
                      n253 = local read "Vname 3"() -> (w929:string)
                    }
                  }
                }
              }
            }
            frame True {
              w931 = u16 2 items=["V", "I", "VPulse", "IPulse", "Common"] ("Mode 2")
              w932 = u16 0 items=["V", "I", "VPulse", "IPulse", "Common"] ("Mode 2")
              n254 = local read "Mode 2"() -> (w933:u16)
              n255 = Equal?(x=w932, y=w933) -> (x = y?=w935:bool)
              n256 = Equal?(x=w933, y=w931) -> (x = y?=w934:bool)
              n257 = Or(x=w935, y=w934) -> (x .or. y?=w930:bool)
              n258 = case shown="True" w930 {
                tunnel: [w938 w939] -> w937
                frame False {
                  n259 = local read "Iname 2"() -> (w938:string)
                }
                frame True {
                  n260 = local read "Vname 2"() -> (w939:string)
                }
              }
            }
          }
        }
        frame True {
          w944 = u16 2 items=["V", "I", "VPulse", "IPulse", "Common"] ("Mode")
          w945 = u16 0 items=["V", "I", "VPulse", "IPulse", "Common"] ("Mode")
          n261 = local read "Mode"() -> (w943:u16)
          n262 = Equal?(x=w943, y=w945) -> (x = y?=w942:bool)
          n263 = Equal?(x=w943, y=w944) -> (x = y?=w941:bool)
          n264 = Or(x=w942, y=w941) -> (x .or. y?=w940:bool)
          n265 = case shown="True" w940 {
            tunnel: [w948 w949] -> w947
            frame False {
              n266 = local read "Iname"() -> (w948:string)
            }
            frame True {
              n267 = local read "Vname"() -> (w949:string)
            }
          }
        }
      }
      n268 = local read "error?"() -> (w576:errorcluster)
      n269 = Unbundle("Y2 axis settings") -> ("Y2 axis on/off"=w568:bool, "MINIMUM"=w581:ext, "MAXIMUM"=w580:ext, "Variable name"=w572:string, "LIN or LOG axis"=w579:string)
      n270 = local read "Var2 step settings"() -> (w591:T3)
      n271 = local read "Var1 sweep settings"() -> (w592:T4)
      n272 = local read "VISA session"() -> (w560:refnum<visa-resource-name>)
      n273 = call "Y1subvi.vi"("MAXIMUM"="MAXIMUM", "Variable name"="Y1 axis", "error in (no error)"=w576, "MINIMUM"="MINIMUM", "LIN or LOG axis"="LIN", "VISA resource name"=w560) -> ("error out"=w577:errorcluster)
      n274 = case shown="False" w568 {
        tunnel: w577 -> [w885 w892]
        tunnel: w560 -> [_ w891]
        tunnel: w581 -> [_ w890]
        tunnel: w580 -> [_ w889]
        tunnel: w572 -> [_ w888]
        tunnel: w579 -> [_ w887]
        tunnel: [w885 w886] -> w578
        frame False {
        }
        frame True {
          n275 = call "Y2subvi.vi"("MAXIMUM"=w889, "Variable name"=w888, "error in (no error)"=w892, "MINIMUM"=w890, "LIN or LOG axis"=w887, "VISA resource name"=w891) -> ("error out"=w886:errorcluster)
        }
      }
      n276 = Unbundle(w591) -> ("total points"=w590:u16)  [unwired: 4 out]
      n277 = Decrement(x=w590) -> (x-1=w550:u16)
      n278 = Unbundle(w592) -> ("start"=w558:dbl)  [unwired: 6 out]
      n279 = call "HP415xA Op-Start-Stop.vi"("error in (no error)"=w578, "function (stop:0)"=w584, "wait until finish"=TRUE, "VISA session"=w560) -> ("error out"=w583:errorcluster)  [unwired: 6 in, 1 out]
      n280 = call "HP415xA Op-Download Trace.vi"("error in (no error)"=w583, "trace (variable) name"=w589, "VISA session"=w560) -> ("error out"=w598:errorcluster, "trace"=w566:dbl[])
      n281 = call "HP415xA Op-Download Trace.vi"("error in (no error)"=w598, "trace (variable) name"="Y1 axis", "VISA session"=w560) -> ("error out"=w573:errorcluster, "trace"=w561:dbl[])
      n282 = case shown="False" w568 {
        tunnel: w573 -> [w870 w878]
        tunnel: w560 -> [_ w877]
        tunnel: w572 -> [_ w876]
        tunnel: [w870 w875] -> w562
        tunnel: w566 -> [w868 w874]
        tunnel: w561 -> [w869 w873]
        tunnel: [w867 w872] -> w569
        tunnel: [dbl[] [] ("trace") w871] -> w567
        frame False {
          n283 = Bundle("trace"=w868, "trace"=w869) -> (w867:cluster{"trace":dbl[], "trace":dbl[]})  [unwired: 1 in]
        }
        frame True {
          n284 = call "HP415xA Op-Download Trace.vi"("error in (no error)"=w878, "trace (variable) name"=w876, "VISA session"=w877) -> ("error out"=w875:errorcluster, "trace"=w871:dbl[])
          n285 = stacked-sequence {
            tunnel: w871 -> [_ w883]
            tunnel: w874 -> [w881 w882]
            tunnel: w873 -> [w880 _]
            tunnel: [w879 _] -> w872
            frame #0 {
              n286 = Bundle("trace"=w881, "trace"=w880) -> (w879:cluster{"trace":dbl[], "trace":dbl[]})  [unwired: 1 in]
            }
            frame #1 {
              n287 = Bundle("trace"=w882, "trace"=w883) -> (→"graphic display 2":cluster{"trace":dbl[], "trace":dbl[]})  [unwired: 1 in]
            }
          }
        }
      }
      "graphic display" <- w569
      n288 = case shown="True" w565 {
        tunnel: w558 -> [_ w737]
        tunnel: w561 -> [w603 w736]
        tunnel: w566 -> [w604 w734]
        tunnel: w550 -> [_ w733]
        tunnel: w560 -> [_ w729]
        tunnel: w562 -> [_ w728]
        tunnel: [w605 w727] -> w564
        tunnel: w559 -> [_ w726]
        tunnel: w559 -> [_ w719]
        tunnel: [dbl[] [] ("trace") w725] -> w563
        tunnel: w557 -> [_ w722]
        tunnel: w556 -> [_ w721]
        tunnel: w555 -> [_ w670]
        tunnel: [_ w644] -> w554
        tunnel: [_ w646] -> w553
        tunnel: w552 -> [_ w687]
        tunnel: w551 -> [_ w686]
        tunnel: w550 -> [_ _]
        tunnel: w549 -> [_ w681]
        frame False {
          n289 = Build Array(w604, w603) -> (w600:dbl[][])
          n290 = local read "error? 2"() -> (w605:errorcluster)
          n291 = call-poly <vilib>:"Write To Spreadsheet File.vi"("transpose? (no:F)"=TRUE ("append to file? (new file:F)"), "format (%.3f)"="%.5e", "2D data"=w600) -> ()  [unwired: 5 in, 1 out]
        }
        frame True {
          w631 = 2
          w632 = 2
          w637 = 1
          w652 = 0
          w650 = 0
          (unwired) 0.000115
          w711 = "%s"
          w660 = "\r"
          n292 = Initialize Array("") -> (w700:string[])  [unwired: 1 in]
          n293 = call "HP415xA Op-Download Trace.vi"("error in (no error)"=w728, "trace (variable) name"=w726, "VISA session"=w729) -> ("error out"=w727:errorcluster, "trace"=w725:dbl[])
          n294 = for {
            N: w733 -> [w793]
            shift-right: [w810] -> w644
            shift-left: w734 -> [w806]
            tunnel: w737 -> [w812]
            tunnel: [w811] -> _ mode=indexing
            shift-right: [w807] -> w646
            shift-left: w736 -> [w809]
            tunnel: [w808] -> w735 mode=indexing
            shift-right: [w803] -> w715
            shift-left: w725 -> [w805]
            tunnel: w719 -> [_]
            tunnel: [w797] -> w717 mode=indexing
            shift-right: [w796] -> w704
            shift-left: w700 -> [w795]
            tunnel: [w793] -> _ mode=indexing
            n295 = Search 1D Array(1D array=w806, element=w812, start index (0)=1) -> (index of element=w804:i32)
            n296 = Split 1D Array(array=w805, index=w804) -> (first subarray=w801:dbl[], second subarray=w803:dbl[])
            n297 = Array Size(array=w801) -> (size(s)=w800:i32)
            n298 = Decrement(x=w800) -> (x-1=w799:i32)
            n299 = Split 1D Array(array=w809, index=w804) -> (first subarray=w808:dbl[], second subarray=w807:dbl[])
            n300 = Split 1D Array(array=w806, index=w804) -> (first subarray=w811:dbl[], second subarray=w810:dbl[])
            n301 = Array Subset(array=w801, index=w799) -> (w802:dbl[])  [unwired: 1 in]
            n302 = Number To Exponential String(number=w802) -> (E-format string=w798:string[])  [unwired: 3 in]
            n303 = Concatenate Strings(w798) -> (w797:string)
            n304 = Build Array (concatenate)("Id", w795) -> (w796:string[])
          }
          n305 = Build Array (concatenate)(w644, w735, w646) -> (w732:dbl[][])
          n306 = Transpose 2D Array(2D array=w732) -> (transposed array=w730:dbl[][])
          n307 = Array To Spreadsheet String(array=w730, 3:"%.5e" ("format string")) -> (spreadsheet string=w720:string)  [unwired: 1 in]
          n308 = local read "Temp (K)"() -> (w624:dbl)
          n309 = Number To Exponential String(number=w624) -> (E-format string=w623:string)  [unwired: 3 in]
          n310 = Build Array("Sample Temp (K):", w623) -> (w622:string[])
          n311 = Build Array("Vg", "Id") -> (w705:string[])
          n312 = Array Size(array=w715) -> (size(s)=w716:i32)
          n313 = Reshape Array(w622, 1 ("start index (0)")) -> (w619:string[])
          n314 = Decrement(x=w716) -> (x-1=w714:i32)
          n315 = Array Subset(array=w715, index=w714) -> (w713:dbl[])  [unwired: 1 in]
          n316 = Insert Into Array(array=w705, index=2, new element=w704) -> (w703:string[])
          n317 = Number To Exponential String(number=w713) -> (E-format string=w709:string[])  [unwired: 3 in]
          n318 = Array To Spreadsheet String(array=w619, 3:"%s") -> (spreadsheet string=w618:string)  [unwired: 1 in]
          n319 = Array To Spreadsheet String(array=w703, 3:w711) -> (spreadsheet string=w710:string)  [unwired: 1 in]
          n320 = Concatenate Strings(w709) -> (w708:string)
          n321 = Build Array (concatenate)("Vd=", w717, w708) -> (w712:string[])
          n322 = Array To Spreadsheet String(array=w712, 3:w711) -> (spreadsheet string=w718:string)  [unwired: 1 in]
          n323 = local read "Vt"() -> (w617:dbl)
          n324 = Fract/Exp String To Number(string="") -> (number=w607:dbl)  [unwired: 3 in, 1 out]
          n325 = Build Array("Mobility (cm^2/Vs):", "On/Off Current:", "Threshold V (V):", "S.T.S. (V/decade):", "Trap Density-VT (Traps/Vcm^2):", "Trap Density-STS (Traps/Vcm^2):") -> (w667:string[])
          n326 = Array Size(array=w644) -> (size(s)=w674:i32)
          n327 = Subtract(x=w674, y="NumPts") -> (x-y=w685:dbl)
          n328 = Initialize Array(0) -> (w684:i32[])  [unwired: 1 in]
          n329 = Initialize Array(w650, w632) -> (w651:i32[])
          n330 = Initialize Array(w650, w632) -> (w649:i32[])
          n331 = Initialize Array(w650) -> (w654:i32[])  [unwired: 1 in]
          n332 = for {
            N: w674 -> [w740]
            shift-right: [w743] -> w673
            shift-left: w646 -> [w744]
            i -> [w739]
            n333 = Subtract(x=w740, y=w739) -> (x-y=w738:i32)
            n334 = Index Array(array=w744, index=w738) -> (element=w741:dbl)
            n335 = Greater Or Equal To 0?(x=w741) -> (x >= 0?=w742:bool)
            n336 = case shown="False" w742 {
              tunnel: w744 -> [w745 w748]
              tunnel: w738 -> [_ w746]
              tunnel: [w745 w747] -> w743
              frame False {
              }
              frame True {
                n337 = Delete From Array(array=w748, index=w746) -> (array with subset deleted=w747:dbl[])  [unwired: 1 in, 1 out]
              }
            }
          }
          n338 = for {
            N: w685 -> [_]
            shift-right: [w787] -> _
            shift-left: w644 -> [w787]
            shift-right: [w788] -> _
            shift-left: w646 -> [w788]
            shift-right: [w792] -> w690
            shift-left: w684 -> [w791]
            shift-right: [w790] -> w688
            shift-left: w654 -> [w789]
            tunnel: "NumPts" -> [w782]
            shift-right: [w778] -> w653
            shift-left: w651 -> [w781]
            shift-right: [w775] -> w642
            shift-left: w649 -> [w776]
            i -> [w779]
            n339 = Array Subset(array=w787, index=w779, length=w782) -> (w777:dbl[])
            n340 = Array Subset(array=w788, index=w779, length=w782) -> (w786:dbl[])
            n341 = Absolute Value(x=w786) -> (abs(x)=w785:dbl[])
            n342 = Build Array (concatenate)(w776, w777) -> (w775:dbl[])
            n343 = Square Root(x=w785) -> (sqrt(x)=w780:dbl[])
            n344 = call <vilib>:"Linear Fit.vi"("Y"=w780, "X"=w777) -> ("Best Linear Fit"=w784:dbl[], "slope"=w774:dbl, "intercept"=w772:dbl)  [unwired: 9 in, 2 out]
            n345 = Insert Into Array(array=w781, index=w779, new element=w780) -> (w778:i32[])
            n346 = call <vilib>:"Goodness of Fit.vi"("Best Fit"=w784, "Y"=w780) -> ("R-square"=w783:dbl)  [unwired: 6 in, 3 out]
            n347 = Negate(x=w774) -> (-x=w773:dbl)
            n348 = Divide(x=w773, y=w772) -> (x/y=w771:dbl)
            n349 = Build Array (concatenate)(w789, w783) -> (w790:dbl[])
            n350 = Build Array (concatenate)(w791, w774) -> (w792:dbl[])
            n351 = local write "Vt"(w771) -> ()
          }
          n352 = Absolute Value(x=w646) -> (abs(x)=w648:dbl[])
          n353 = Array Max & Min(array=w673) -> (max value=w671:dbl, min value=w672:dbl)  [unwired: 2 out]
          n354 = Square Root(x=w648) -> (sqrt(x)=w647:dbl[])
          n355 = Initialize Array(w652, w631) -> (w641:i32[])
          n356 = Initialize Array(w652, w631) -> (w659:i32[])
          n357 = Divide(x=w672, y=w671) -> (x/y=w609:dbl)
          n358 = for {
            N: 20 -> [_]
            shift-right: [w769] -> _
            shift-left: w688 -> [w770]
            shift-right: [w761] -> _
            shift-left: w690 -> [w759]
            shift-right: [w760] -> w691
            shift-left: w659 -> [w768]
            shift-right: [w767] -> w682
            shift-left: w659 -> [w766]
            shift-right: [w757] -> _
            shift-left: w653 -> [w758]
            shift-right: [w756] -> w640
            shift-left: w641 -> [w764]
            shift-right: [w749] -> _
            shift-left: w642 -> [w751]
            shift-right: [w753] -> w639
            shift-left: w641 -> [w752]
            w755 = 1
            n359 = Array Max & Min(array=w770) -> (max value=w765:dbl, max index (indices)=w750:i32)  [unwired: 2 out]
            n360 = Array Subset(array=w751, index=w750, length=w755) -> (w754:dbl[])
            n361 = Array Subset(array=w758, index=w750, length=w755) -> (w763:i32[])
            n362 = Array Subset(array=w759, index=w750, length=w755) -> (w762:dbl[])
            n363 = Build Array (concatenate)(w768, w762) -> (w760:dbl[])
            n364 = Delete From Array(array=w770, index=w750) -> (array with subset deleted=w769:dbl[])  [unwired: 1 in, 1 out]
            n365 = Build Array (concatenate)(w752, w754) -> (w753:dbl[])
            n366 = Build Array (concatenate)(w766, w765) -> (w767:dbl[])
            n367 = Build Array (concatenate)(w764, w763) -> (w756:i32[])
            n368 = Delete From Array(array=w758, index=w750) -> (array with subset deleted=w757:i32[])  [unwired: 1 in, 1 out]
            n369 = Delete From Array(array=w751, index=w750) -> (array with subset deleted=w749:dbl[])  [unwired: 1 in, 1 out]
            n370 = Delete From Array(array=w759, index=w750) -> (array with subset deleted=w761:dbl[])  [unwired: 1 in, 1 out]
          }
          "Max R" <- w682
          n371 = local write "On/Off Current"(w609) -> ()
          n372 = Bundle("trace"=w644, w647) -> (w645:cluster{"trace":dbl[], dbl[]})  [unwired: 1 in]
          n373 = Fract/Exp String To Number(string=w687) -> (number=w657:dbl)  [unwired: 3 in, 1 out]
          n374 = local read "Vt"() -> (w616:dbl)
          n375 = Fract/Exp String To Number(string=w686) -> (number=w658:dbl)  [unwired: 3 in, 1 out]
          n376 = Fract/Exp String To Number(string=w681) -> (number=w676:dbl)  [unwired: 3 in, 1 out]
          n377 = Array Max & Min(array=w691) -> (min value=w633:dbl, min index (indices)=w634:i32)  [unwired: 2 out]
          n378 = Array Subset(array=w639, index=w634, length=w637) -> (w635:dbl[])
          n379 = Array Subset(array=w640, index=w634, length=w637) -> (w638:i32[])
          n380 = Bundle(w635, w638) -> (w636:cluster{dbl[], i32[]})  [unwired: 1 in]
          n381 = Build Array(w645, w636) -> (→"XY Graph":cluster{"trace":dbl[], dbl[]}[])
          n382 = Absolute Value(x=w616) -> (abs(x)=w615:dbl)
          n383 = Square(x=w633) -> (x^2=w692:dbl)
          n384 = Multiply(x=2, y=w692) -> (x*y=w693:dbl)
          n385 = Multiply(x=3.9, y=8.854e-12) -> (x*y=w678:dbl)
          n386 = Multiply(x=w658, y=w693) -> (x*y=w694:dbl)
          n387 = Multiply(x=w676, y=1e-09) -> (x*y=w675:dbl)
          n388 = Divide(x=w678, y=w675) -> (x/y=w614:dbl)
          n389 = Multiply(x=w615, y=w614) -> (x*y=w613:dbl)
          n390 = Divide(x=w613, y=1.602e-19) -> (x/y=w610:dbl)
          n391 = Multiply(x=w657, y=w614) -> (x*y=w695:dbl)
          n392 = Divide(x=w694, y=w695) -> (x/y=w697:dbl)
          n393 = Multiply(x=w697, y=10000) -> (x*y=w611:dbl)
          n394 = Build Array(w611, w609, w617, w607, w610, w607) -> (w666:dbl[])
          n395 = Number To Exponential String(number=w666) -> (E-format string=w665:string[])  [unwired: 3 in]
          n396 = Build Array(w667, w665) -> (w664:string[][])
          n397 = Transpose 2D Array(2D array=w664) -> (transposed array=w663:string[][])
          n398 = Array To Spreadsheet String(array=w663, 3:"%s") -> (spreadsheet string=w661:string)  [unwired: 1 in]
          n399 = Concatenate Strings(w722, w660, w721, w660, w670, w618, w660, w661, w660, w718, w710, w720, "\r") -> (w724:string)
          n400 = call <vilib>:"Write Characters To File.vi"("append to file? (new file:F)"=TRUE, "character string"=w724, "file path (dialog if empty)"="Input Path") -> ("new file path (Not A Path if cancelled)"=w606:path)  [unwired: 2 in]
          n401 = local write "Output Path"(w606) -> ()
          n402 = local write "Trap Density-VT"(w610) -> ()
          n403 = local write "Mobility"(w611) -> ()
        }
      }
      n404 = case shown="True" w568 {
        tunnel: w550 -> [_ w819]
        tunnel: w565 -> [_ w820]
        tunnel: w566 -> [_ w818]
        tunnel: w558 -> [_ w817]
        tunnel: w567 -> [_ w816]
        tunnel: w563 -> [_ w815]
        tunnel: w559 -> [_ w814]
        frame False {
        }
        frame True {
          n405 = case shown="True" w820 {
            tunnel: w819 -> [_ w836]
            tunnel: w818 -> [w824 w851]
            tunnel: w817 -> [_ w850]
            tunnel: w816 -> [w825 w849]
            tunnel: w815 -> [_ w848]
            tunnel: w814 -> [_ w831]
            frame False {
              n406 = Build Array(w824, w825) -> (w823:dbl[][])
              n407 = call-poly <vilib>:"Write To Spreadsheet File.vi"("transpose? (no:F)"=TRUE, "format (%.3f)"="%.5e", "2D data"=w823) -> ()  [unwired: 5 in, 1 out]
            }
            frame True {
              n408 = for {
                N: w836 -> [_]
                shift-right: [w862] -> w847
                shift-left: w851 -> [w863]
                tunnel: w850 -> [w865]
                tunnel: [w861] -> _ mode=indexing
                shift-right: [w858] -> w845
                shift-left: w849 -> [w860]
                tunnel: [w859] -> w846 mode=indexing
                shift-right: [w855] -> w840
                shift-left: w848 -> [w856]
                tunnel: [w852] -> w837 mode=indexing
                n409 = Search 1D Array(1D array=w863, element=w865, start index (0)=1) -> (index of element=w857:i32)
                n410 = Split 1D Array(array=w863, index=w857) -> (first subarray=w861:dbl[], second subarray=w862:dbl[])
                n411 = Split 1D Array(array=w860, index=w857) -> (first subarray=w859:dbl[], second subarray=w858:dbl[])
                n412 = Split 1D Array(array=w856, index=w857) -> (first subarray=w853:dbl[], second subarray=w855:dbl[])
                n413 = Index Array(array=w853, index=1) -> (element=w852:dbl)
              }
              n414 = Build Array (concatenate)(w847, w846, w845) -> (w844:dbl[][])
              n415 = Index Array(array=w840, index=1) -> (element=w838:dbl)
              n416 = Transpose 2D Array(2D array=w844) -> (transposed array=w843:dbl[][])
              n417 = Insert Into Array(array=w837, index=w836, new element=w838) -> (w835:dbl[])
              n418 = Array To Spreadsheet String(delimiter (Tab)=",", array=w835, 3:"%.5e" ("format string")) -> (spreadsheet string=w829:string)
              n419 = Array To Spreadsheet String(delimiter (Tab)=",", array=w843, 3:"%.5e" ("format string")) -> (spreadsheet string=w827:string)
              n420 = Concatenate Strings(w831, "," ("string")) -> (w830:string)
              n421 = Concatenate Strings(w830, w829) -> (w828:string)
              n422 = Concatenate Strings(w828, w827) -> (w826:string)
              n423 = call <vilib>:"Write Characters To File.vi"("character string"=w826) -> ()  [unwired: 4 in, 1 out]
            }
          }
        }
      }
      n424 = call "HP415xA Sys-Error Query.vi"("VISA session"=w560, "error in (no error)"=w564) -> ("error out"=w596:errorcluster)  [unwired: 2 in, 1 out]
      n425 = call "HP415xA  Close.vi"("error in (no error)"=w596, "VISA session"=w560) -> ("error out"=w597:errorcluster)
      n426 = local write "error?"(w597) -> ()
    }
    frame #6 {
      n427 = flat-sequence {
        frame #0 {
          n428 = local read "Output Path"() -> (w982:path)
          n429 = local read "Sample Properties:"() -> (w978:T1)
          n430 = local read "Temp (K)"() -> (w969:dbl)
          n431 = call "sub_thresh_swing_subvi.vi"("Path"=w982) -> ("Sub Threshold Swing"=w968:dbl)  [unwired: 10 in, 4 out]
          n432 = Unbundle By Name(w978) -> ("SiO2 Thickness"=w971:string)
          n433 = Equal To 0?(x=w969) -> (x = 0?=w981:bool)
          n434 = local write "STS"(w968) -> ()
          n435 = case shown="True" w981 {
            tunnel: [w983 290] -> w980
            tunnel: w969 -> [w983 _]
            frame False {
            }
            frame True {
            }
          }
          n436 = Fract/Exp String To Number(string=w971) -> (number=w973:dbl)  [unwired: 3 in, 1 out]
          n437 = Multiply(x=3.9, y=8.854e-12) -> (x*y=w977:dbl)
          n438 = Multiply(x=w973, y=1e-09) -> (x*y=w974:dbl)
          n439 = Divide(x=w977, y=w974) -> (x/y=w970:dbl)
          n440 = call "Trap Density_STS.vi"("Temp (T) [K]"=w980, "S.T.S. (S)"=w968, "Dielectric"=w970) -> ("Trap Density (N)"=w979:dbl)  [unwired: 8 in]
          n441 = local write "Trap Density-STS"(w979) -> ()
        }
        frame #1 {
          n442 = local read "Output Path"() -> (w985:path)
          n443 = call-poly <vilib>:"Read From Spreadsheet File.vi"("file path (dialog if empty)"=w985) -> ("all rows"=w992:string[][])  [unwired: 6 in, 4 out]
          n444 = Array Subset(array=w992, index (col)=0, length (col)=1) -> (w1000:string[][])  [unwired: 2 in]
          n445 = Reshape Array(w1000, 100) -> (w997:string[])
          n446 = Search 1D Array(1D array=w997, element="S.T.S. (V/decade):") -> (index of element=w995:i32)  [unwired: 1 in]
          n447 = Search 1D Array(1D array=w997, element="Trap Density-STS (Traps/Vcm^2):") -> (index of element=w989:i32)  [unwired: 1 in]
          n448 = local read "Trap Density-STS"() -> (w988:dbl)
          n449 = local read "STS"() -> (w996:dbl)
          n450 = Number To Exponential String(number=w996) -> (E-format string=w993:string)  [unwired: 3 in]
          n451 = Replace Array Subset(array=w992, new element=w993, index (row)=w995, index (col)=1) -> (w991:string[][])
          n452 = Number To Exponential String(number=w988) -> (E-format string=w987:string)  [unwired: 3 in]
          n453 = Replace Array Subset(array=w991, new element=w987, index (row)=w989, index (col)=1) -> (w986:string[][])
          "Array" <- w986
          n454 = call-poly <vilib>:"Write To Spreadsheet File.vi"("2D data"=w986, "file path (dialog if empty)"=w985) -> ()  [unwired: 6 in, 1 out]
        }
      }
    }
  }
